vi "UpdatePluginIndex.vi"(8 "Error":errorcluster[](array[cluster]), 9 "Index":u32, 10 "PluginName":string, 11 "Test":refnum<class "Test.lvclass">) -> (0 "Error":errorcluster[](array[cluster]), 3 "Test":refnum<class "Test.lvclass">)   [LabVIEW 2018, in "Test.lvclass"]
uses:
  Test.lvclass
  Test.lvclass/Test.ctl
  Accessors/Read PluginIndex.vi
  Accessors/Write PluginIndex.vi
  <userlib>/NIST/NISTErrorLib/NISTErrorLib.lvlib
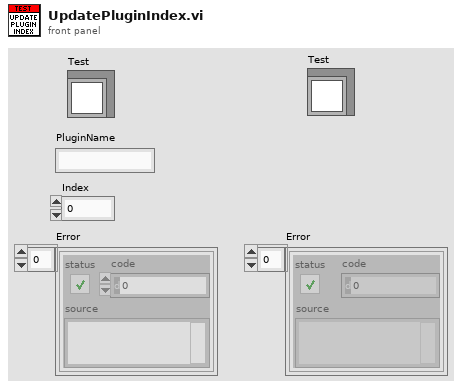
[diagram p1: front panel]
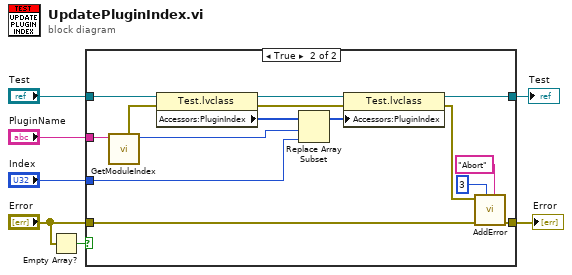
[diagram p0: block diagram]
diagram:
  n1 = Empty Array?(array="Error") -> (empty?=w7:bool)
  n2 = case shown="True" w7 {
    tunnel: "Error" -> [w9 w14]
    tunnel: [w9 w13] -> w5
    tunnel: "Test" -> [w8 w23]
    tunnel: "PluginName" -> [_ w24]
    tunnel: "Index" -> [_ w20]
    tunnel: [w8 w17] -> w1
    frame False {
    }
    frame True {
      n3 = call "GetModuleIndex.vi"("ModuleType"=w24) -> ("ModuleIndex"=w21:i32, "Error"=w16:errorcluster)  [unwired: 9 in]
      n4 = property class="Test.lvclass"(reference=w23, error in=w16) -> (reference out=w19:refnum<class "Test.lvclass">, error out=w15:errorcluster, "Accessors:PluginIndex"=w22:u32[])
      n5 = Replace Array Subset(array=w22, new element=w20, index=w21) -> (w18:u32[])
      n6 = property class="Test.lvclass"(reference=w19, error in=w15, "Accessors:PluginIndex"=w18) -> (reference out=w17:refnum<class "Test.lvclass">, error out=w12:errorcluster)
      n7 = call <userlib>:"AddError.vi"("Severity"="Abort", "Priority"=u8 3, "ErrorArray"=w14, "error in (no error)"=w12) -> ("ErrorArray"=w13:errorcluster[])  [unwired: 6 in, 1 out]
    }
  }
  "Test" <- w1
  "Error" <- w5
